vi "Add Message to Bus Controller.vi"(4 "create timestamp channel":bool, 5 "status channels directions":enum16{"Rx", "Tx", "Unspecified"}[](array[ring])=[enum."Unspecified"], 6 "parameters":T3(array[cluster]), 7 "number of words":u16, 8 "error in":errorcluster, 9 "direction":T4, 10 "name":string, 11 "port":T1 format="%.0x") -> (0 "error out":errorcluster, 2 "message":T1=18446744073709551615 format="%.0x", 3 "port out":T1 format="%.0x")   [LabVIEW 2020, in "AIM MIL-STD-1553 Scripting.lvlib"]
doc: "Adds a new <b>message</b> with the specified <b>name</b> to the Bus Controller of the specified <b>port</b>. Then performs the following in the Message Section:\n1. Adds a Message Status Channel for each of the values in <b>status channels directions</b>.\n2. Sets the <b>number of words</b> property for the Message Section.\n3. Adds a Parameter Channel with the specified <b>direction</b> for each item in <b>parameters</b>.\n4. Creates a Timestamp channel if <b>create timestamp channel</b> is True."
uses:
  AIM MIL-STD-1553 Scripting.lvlib
  Shared/Direction.ctl
  Shared/Parameter Definition.ctl
  <vilib>/NI VeriStand/Custom Device API/Custom Device Item Ref.ctl
  <vilib>/NI VeriStand/Custom Device API/Custom Device API.lvlib
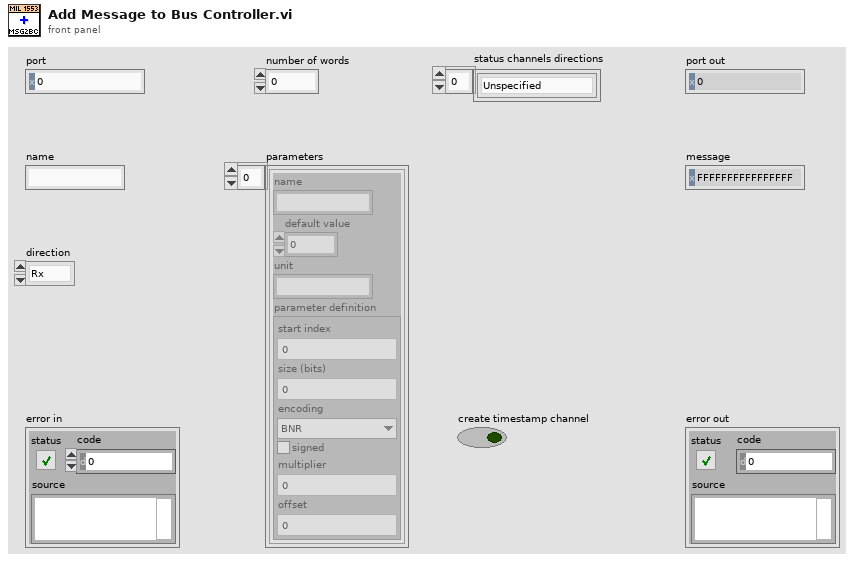
[diagram p1: front panel]
types:
  T1 = typedef "Custom Device API.lvlib/Custom Device Item Ref.ctl" = u64
  T2 = typedef "Parameter Definition.ctl" = cluster{"start index":i32, "size (bits)":i32, "encoding":enum16{"BNR", "BCD", "Discrete"}, "signed":bool, "multiplier":dbl, "offset":dbl}
  T3 = cluster{"name":string, "default value":dbl, "unit":string, "parameter definition":T2}[]
  T4 = typedef "Direction.ctl" = enum16{"Rx", "Tx"}
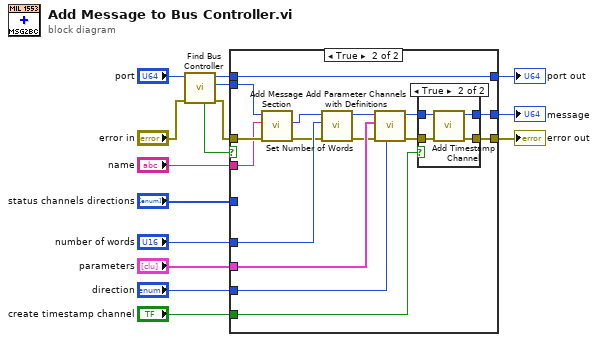
[diagram p0: block diagram]
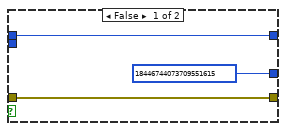
[diagram p2: hidden frame]
diagram:
  n1 = call "Find Bus Controller.vi"("error in"="error in", "port"="port") -> ("error out"=w7:errorcluster, "bus controller"=w6:T1, "port out"=w5:T1, "found?"=w4:bool)  [unwired: 6 in]
  n2 = case shown="True" w4 {
    tunnel: w5 -> [w18 w25]
    tunnel: w6 -> [_ w33]
    tunnel: w7 -> [w17 w34]
    tunnel: [w17 w23] -> w8
    tunnel: [w18 w25] -> w9
    tunnel: "number of words" -> [_ w32]
    tunnel: "parameters" -> [_ w31]
    tunnel: "name" -> [_ w28]
    tunnel: "direction" -> [_ w27]
    tunnel: "create timestamp channel" -> [_ w26]
    tunnel: "status channels directions" -> [_ _]
    tunnel: [T1 18446744073709551615 ("message out") w21] -> w1
    frame False {
    }
    frame True {
      n3 = call "Add Message Section.vi"("error in"=w34, "message section name"=w28, "bus controller"=w33) -> ("error out"=w20:errorcluster, "message section"=w19:T1)  [unwired: 6 in, 1 out]
      n4 = call "Set Number of Words.vi"("error in"=w20, "number of words"=w32, "message or subaddress"=w19) -> ("error out"=w29:errorcluster, "message or subaddress out"=w30:T1)  [unwired: 7 in]
      n5 = call "Add Parameter Channels with Definitions.vi"("direction"=w27, "error in"=w29, "parameters"=w31, "message or subaddress"=w30) -> ("error out"=w24:errorcluster, "message or subaddress out"=w22:T1)  [unwired: 6 in]
      n6 = case shown="True" w26 {
        tunnel: w24 -> [w36 w40]
        tunnel: w22 -> [w35 w39]
        tunnel: [w36 w38] -> w23
        tunnel: [w35 w37] -> w21
        frame False {
        }
        frame True {
          n7 = call "Add Timestamp Channel.vi"("error in"=w40, "message section"=w39) -> ("error out"=w38:errorcluster, "message section out"=w37:T1)  [unwired: 7 in, 1 out]
        }
      }
    }
  }
  "port out" <- w9
  "error out" <- w8
  "message" <- w1
